vi "Auto Balance Loop.vi"(2 "error in (no error)":errorcluster, 3 "LBCB Number":T1) -> (0 "error out":errorcluster)   [LabVIEW 2009]
uses:
  lib/Data Access Objects/Metadata/LBCB Number.ctl
  Update Actions.ctl
  lib/Data Access Objects/Metadata/Persistant DAO Actions.ctl
panel:
  in  "L2 Default Balance Gain":dbl[](array[numeric])=[0.05, 0.05, 0.05, 0.05, 0.05, 0.05] caption="Balance Gain\n(V/V)"
  in  "L2 Default Safe Range":dbl[](array[numeric])=[0.02, 0.02, 0.02, 0.02, 0.02, 0.02] caption="Safe Range\n(V)"
  in  "L1 Default Balance Gain":dbl[](array[numeric])=[0.05, 0.05, 0.05, 0.05, 0.05, 0.05] caption="Balance Gain\n(V/V)"
  in  "L1 Default Safe Range":dbl[](array[numeric])=[0.02, 0.02, 0.02, 0.02, 0.02, 0.02] caption="Safe Range\n(V)"
  in  "Cancel":bool
  in  "OK":bool
  in  "Safe Range":dbl[](array[numeric])=[0.02, 0.02, 0.02, 0.02, 0.02, 0.02] caption="Safe Range\n(V)"
  # "Auto Balance Feedback Loop Properties"
  # "Actuator X1"
  # "Actuator X2"
  # "Actuator Y1"
  # "Actuator Z1"
  # "Actuator Z2"
  # "Actuator Z3"
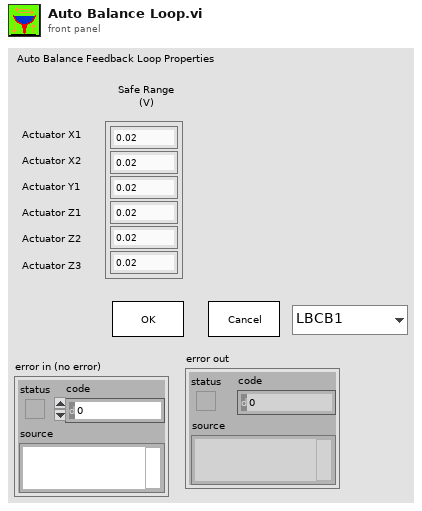
[diagram p1: front panel]
types:
  T1 = typedef "LBCB Number.ctl" = enum16{"LBCB1", "LBCB2"}
  T2 = typedef "Persistant DAO Actions.ctl" = enum16{"Init", "Get", "Set", "Load", "Save"}
  T3 = typedef "Update Actions.ctl" = enum16{"Update", "Exit"}
  T4 = typedef "Actuator Point.ctl" = cluster{"X1":dbl, "X2":dbl, "Y1":dbl, "Z1":dbl, "Z2":dbl, "Z3":dbl}
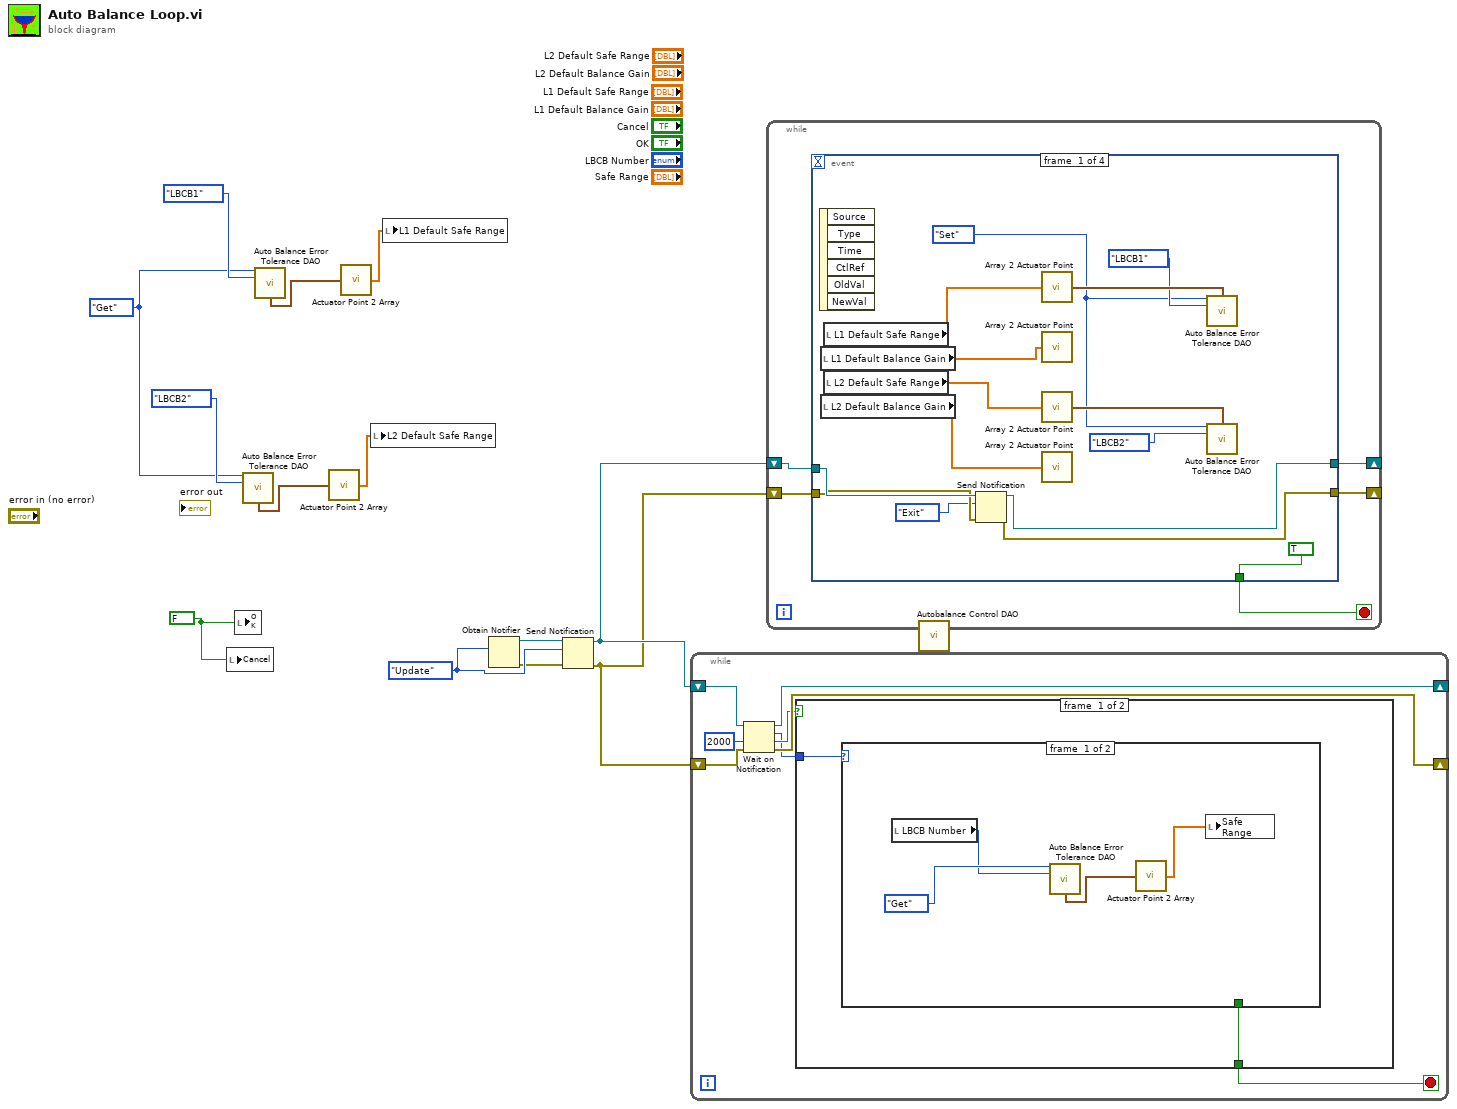
[diagram p0: block diagram]
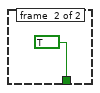
[diagram p2: hidden frame]
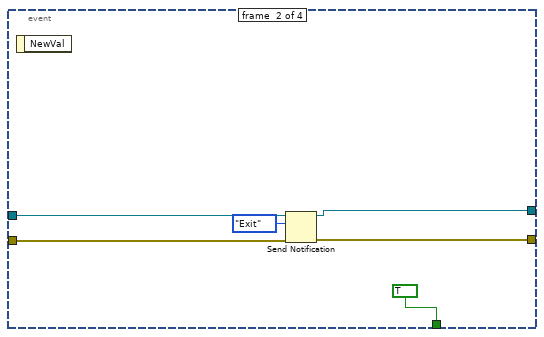
[diagram p4: hidden frame]
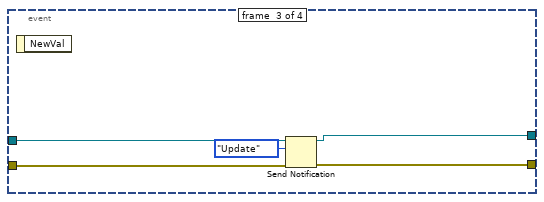
[diagram p5: hidden frame]
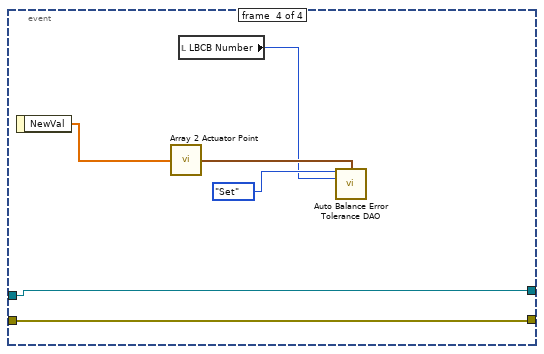
[diagram p6: hidden frame]
diagram:
  w1 = FALSE
  w4 = Persistant_DAO_Actions."Get" ("Auto Balance Increment Actions")
  w13 = Update_Actions."Update" ("Update Actions")
  n1 = local write "Cancel"(w1) -> ()
  n2 = local write "OK"(w1) -> ()
  n3 = call "Auto Balance Error Tolerance DAO.vi"("Auto Balance Increment Actions"=w4, "LBCB Number"=LBCB_Number."LBCB2") -> ("Auto Balance Error Out"=w7:T4)  [unwired: 3 in, 10 out]
  n4 = call "Auto Balance Error Tolerance DAO.vi"("Auto Balance Increment Actions"=w4, "LBCB Number"=LBCB_Number."LBCB1") -> ("Auto Balance Error Out"=w10:T4)  [unwired: 3 in, 10 out]
  n5 = call "Actuator Point 2 Array.vi"("Actuator Point"=w7) -> ("Array"=w6:dbl[])
  n6 = call "Actuator Point 2 Array.vi"("Actuator Point"=w10) -> ("Array"=w9:dbl[])
  n7 = local write "L2 Default Safe Range"(w6) -> ()
  n8 = local write "L1 Default Safe Range"(w9) -> ()
  n9 = Obtain Notifier(notification data type=w13) -> (notifier out=w12:refnum<notifier>, error out=w11:errorcluster)  [unwired: 2 in, 2 out]
  n10 = Send Notification(notification=w13, notifier=w12, error in (no error)=w11) -> (notifier out=w3:refnum<notifier>, error out=w2:errorcluster)
  n11 = while {
    shift-right: [w19] -> _
    shift-left: w3 -> [w20]
    shift-right: [w18] -> _
    shift-left: w2 -> [w21]
    stop <- w15 stop-if-true
    n12 = Wait on Notification(notifier=w20, timeout in ms (-1)=2000, error in (no error)=w21) -> (notifier out=w19:refnum<notifier>, notification=w16:T3, timed out?=w17:bool, error out=w18:errorcluster)  [unwired: 1 out]
    n13 = case shown="False" w17 {
      tunnel: w16 -> [w23 _]
      tunnel: [w22 _] -> w15
      frame #0 {
        n14 = case shown="\"Update\"" w23 {
          tunnel: [_ TRUE] -> w22
          frame #0 {
            n15 = local read "LBCB Number"() -> (w24:T1)
            n16 = call "Auto Balance Error Tolerance DAO.vi"("Auto Balance Increment Actions"=Persistant_DAO_Actions."Get", "LBCB Number"=w24) -> ("Auto Balance Error Out"=w26:T4)  [unwired: 3 in, 10 out]
            n17 = call "Actuator Point 2 Array.vi"("Actuator Point"=w26) -> ("Array"=w25:dbl[])
            n18 = local write "Safe Range"(w25) -> ()
          }
          frame #1 {
          }
        }
      }
      frame #1 {
      }
    }
  }
  n19 = while {
    shift-right: [w30] -> _
    shift-left: w3 -> [w32]
    shift-right: [w29] -> _
    shift-left: w2 -> [w31]
    stop <- w33 stop-if-true
    n20 = event shown="[3] \"Safe Range\": Value Change" {
      selector: _ -> [_ _ _ _]
      dyn-events: _ -> [_ _ _ _]
      timeout: _ -> [_ _ _ _]
      tunnel: [TRUE TRUE _ _] -> w33
      tunnel: w32 -> [w38 w53 w59 w61]
      tunnel: w31 -> [w37 w52 w58 w60]
      tunnel: [w35 w50 w56 w61] -> w30
      tunnel: [w34 w49 w55 w60] -> w29
      event #0 {
        w41 = Persistant_DAO_Actions."Set" ("Auto Balance Increment Actions")
        n21 = event-data() -> ()  [unwired: 7 out]
        n22 = local read "L1 Default Balance Gain"() -> (w44:dbl[])
        n23 = local read "L2 Default Balance Gain"() -> (w39:dbl[])
        n24 = local read "L1 Default Safe Range"() -> (w45:dbl[])
        n25 = local read "L2 Default Safe Range"() -> (w40:dbl[])
        n26 = Send Notification(notification=Update_Actions."Exit", notifier=w38, error in (no error)=w37) -> (notifier out=w35:refnum<notifier>, error out=w34:errorcluster)
        n27 = call "Array 2 Actuator Point.vi"("Array"=w45) -> ("Actuator Point"=w48:T4)
        n28 = call "Array 2 Actuator Point.vi"("Array"=w44) -> ()  [unwired: 1 out]
        n29 = call "Array 2 Actuator Point.vi"("Array"=w40) -> ("Actuator Point"=w42:T4)
        n30 = call "Array 2 Actuator Point.vi"("Array"=w39) -> ()  [unwired: 1 out]
        n31 = call "Auto Balance Error Tolerance DAO.vi"("Auto Balance Increment Actions"=w41, "Auto Balance Error In"=w48, "LBCB Number"=LBCB_Number."LBCB1") -> ()  [unwired: 2 in, 11 out]
        n32 = call "Auto Balance Error Tolerance DAO.vi"("Auto Balance Increment Actions"=w41, "Auto Balance Error In"=w42, "LBCB Number"=LBCB_Number."LBCB2") -> ()  [unwired: 2 in, 11 out]
      }
      event #1 {
        n33 = event-data() -> ()  [unwired: 2 out]
        n34 = Send Notification(notification=Update_Actions."Exit", notifier=w53, error in (no error)=w52) -> (notifier out=w50:refnum<notifier>, error out=w49:errorcluster)
      }
      event #2 {
        n35 = event-data() -> ()  [unwired: 2 out]
        n36 = Send Notification(notification=Update_Actions."Update", notifier=w59, error in (no error)=w58) -> (notifier out=w56:refnum<notifier>, error out=w55:errorcluster)
      }
      event #3 {
        n37 = event-data() -> ("NewVal"=w62:dbl[])  [unwired: 1 out]
        n38 = call "Array 2 Actuator Point.vi"("Array"=w62) -> ("Actuator Point"=w65:T4)
        n39 = local read "LBCB Number"() -> (w63:T1)
        n40 = call "Auto Balance Error Tolerance DAO.vi"("Auto Balance Increment Actions"=Persistant_DAO_Actions."Set", "Auto Balance Error In"=w65, "LBCB Number"=w63) -> ()  [unwired: 2 in, 11 out]
      }
    }
  }
  n41 = call "Autobalance Control DAO.vi"() -> ()  [unwired: 4 in, 8 out]
